vi "TCL Event Viewer.vi"() -> ()   [LabVIEW 2010]
uses:
  <vilib>/Utility/file.llb/Read From Spreadsheet File (string).vi
  TCL Select Fragments/TCL Select Fragments NfragsNcriteria.vi
panel:
  in  "load":bool
  in  "save":bool
  out "event":string
  in  "pick baseline":bool
  in  "auto baseline":bool=TRUE
  in  "load defaults":bool
  in  "calibration constant":dbl=1.0 step=0.0001 format="%#_9f"
  in  "ignore fraction":dbl=0.1875 min=0.0 max=1.0 step=0.0001
  in  "fit fraction":dbl=0.18 min=0.0 max=1.0 step=0.0001
  in  "ignore first":i32=5 min=0 step=1
  in  "subtract fraction":dbl=0.125 min=0.0 max=1.0 step=0.0001
  out "busy":bool
  in  "show all events":bool
  in  "stop":bool
  out "error out":errorcluster
  in  "error in (no error)":errorcluster
  out "polarization %":dbl
  out "area":dbl
  in  "fit order":i32=3 min=0 step=1
  out "fit coefficients":dbl[](array[numeric])
  out "baseline time":timestamp format="%<%H:%M:%S\n%x>T"
  out "baseline":string
  out "raw plot":cluster{dbl[], "signal":dbl[]}[](graph)
  out "poly plot":cluster{dbl[], "poly fit":dbl[]}[](graph)
  out "signal plot":cluster{dbl[], "signal":dbl[]}(graph)
  in  "events list":i32(listbox)
  in  "y axis":string(combo)
  out "events plot":cluster{timestamp, dbl}[](graph)
  out "raw data":string[][](table)
  in  "auto advance":bool
  in  "real time":bool
  in  "end time":timestamp format="%<%H:%M:%S\n%x>T"
  in  "start time":timestamp format="%<%H:%M:%S\n%x>T"
  in  "filter":T1(array[cluster])
  in  "pick baseline files":bool
  in  "use current event file":bool
  in  "pick event files":bool
  in  "additional baseline files":path[](array[path])
  in  "event files":path[](array[path])
  # "Do not operate panel while busy light is on"
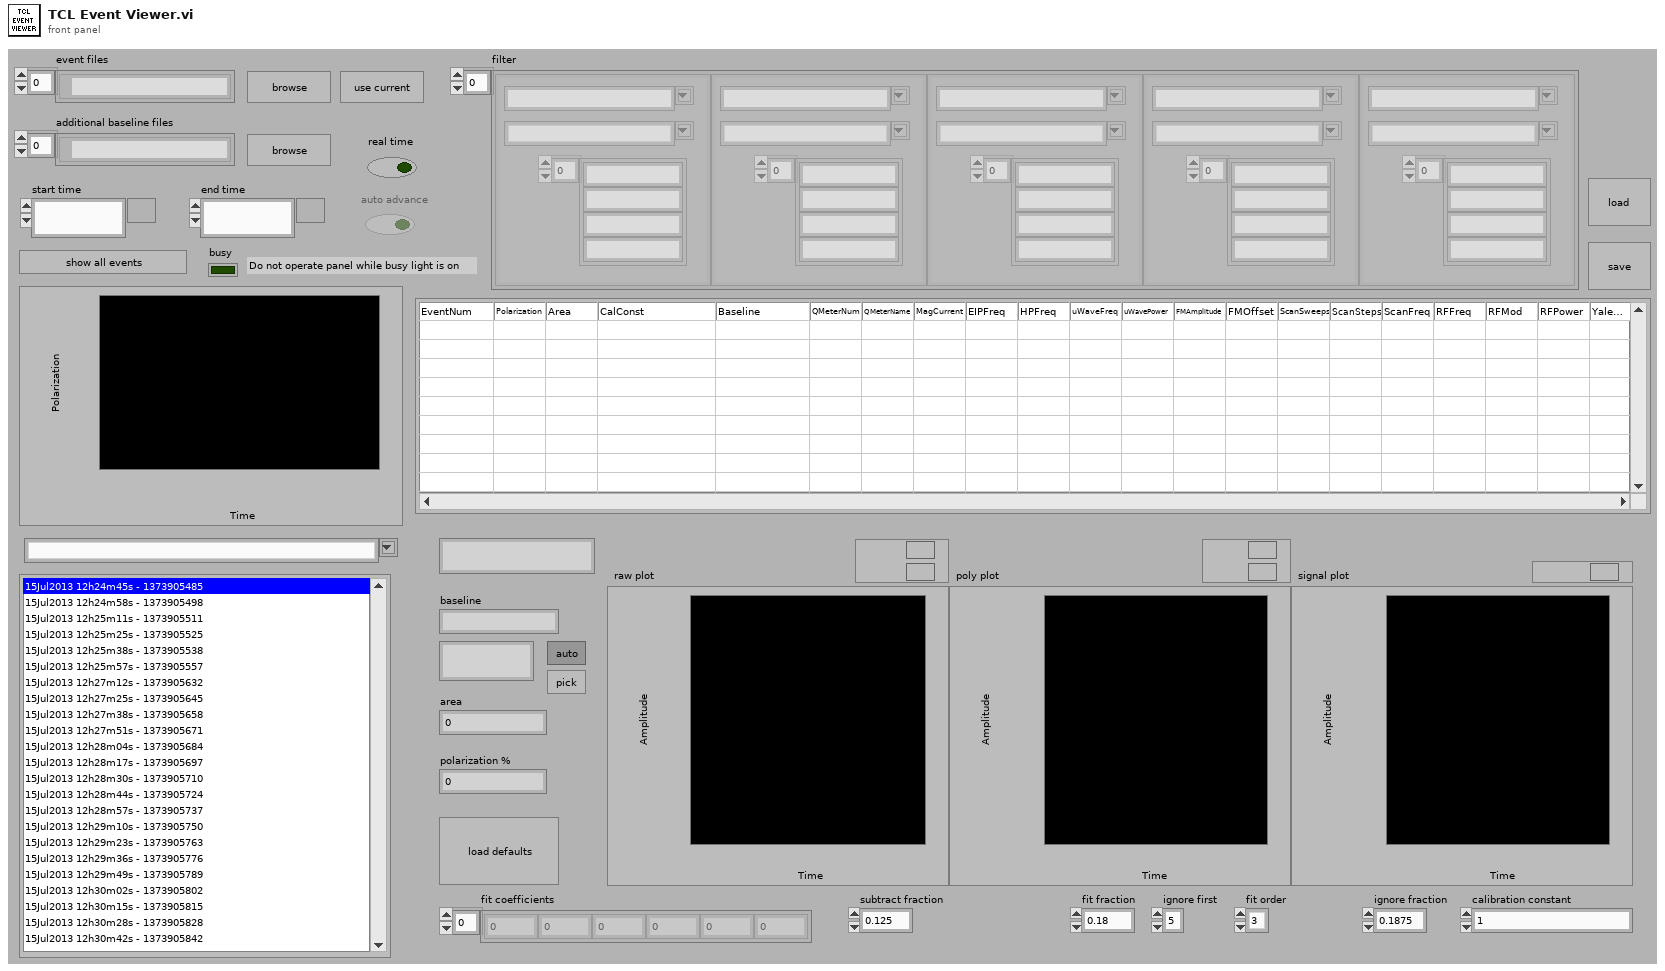
[diagram p1: front panel]
types:
  T1 = cluster{"fragment":string, "criteria":string[], "operator":string}[]
  T2 = enum16{"idle", "import events", "filter events", "plot events", "read plot data", "plot signals"}
  T3 = enum16{"idle", "import events", "filter events", "plot events", "plot signals"}
  T4 = cluster{"primary key":string, "criteria":string[], "operator":string}[]
  T5 = enum16{"big-endian, network order", "native, host order", "little-endian"}
  T6 = cluster{"fragment":string, "criteria":string[], "operator":string}
  T7 = enum8{"Enabled", "Disabled", "Disabled and Grayed Out"}
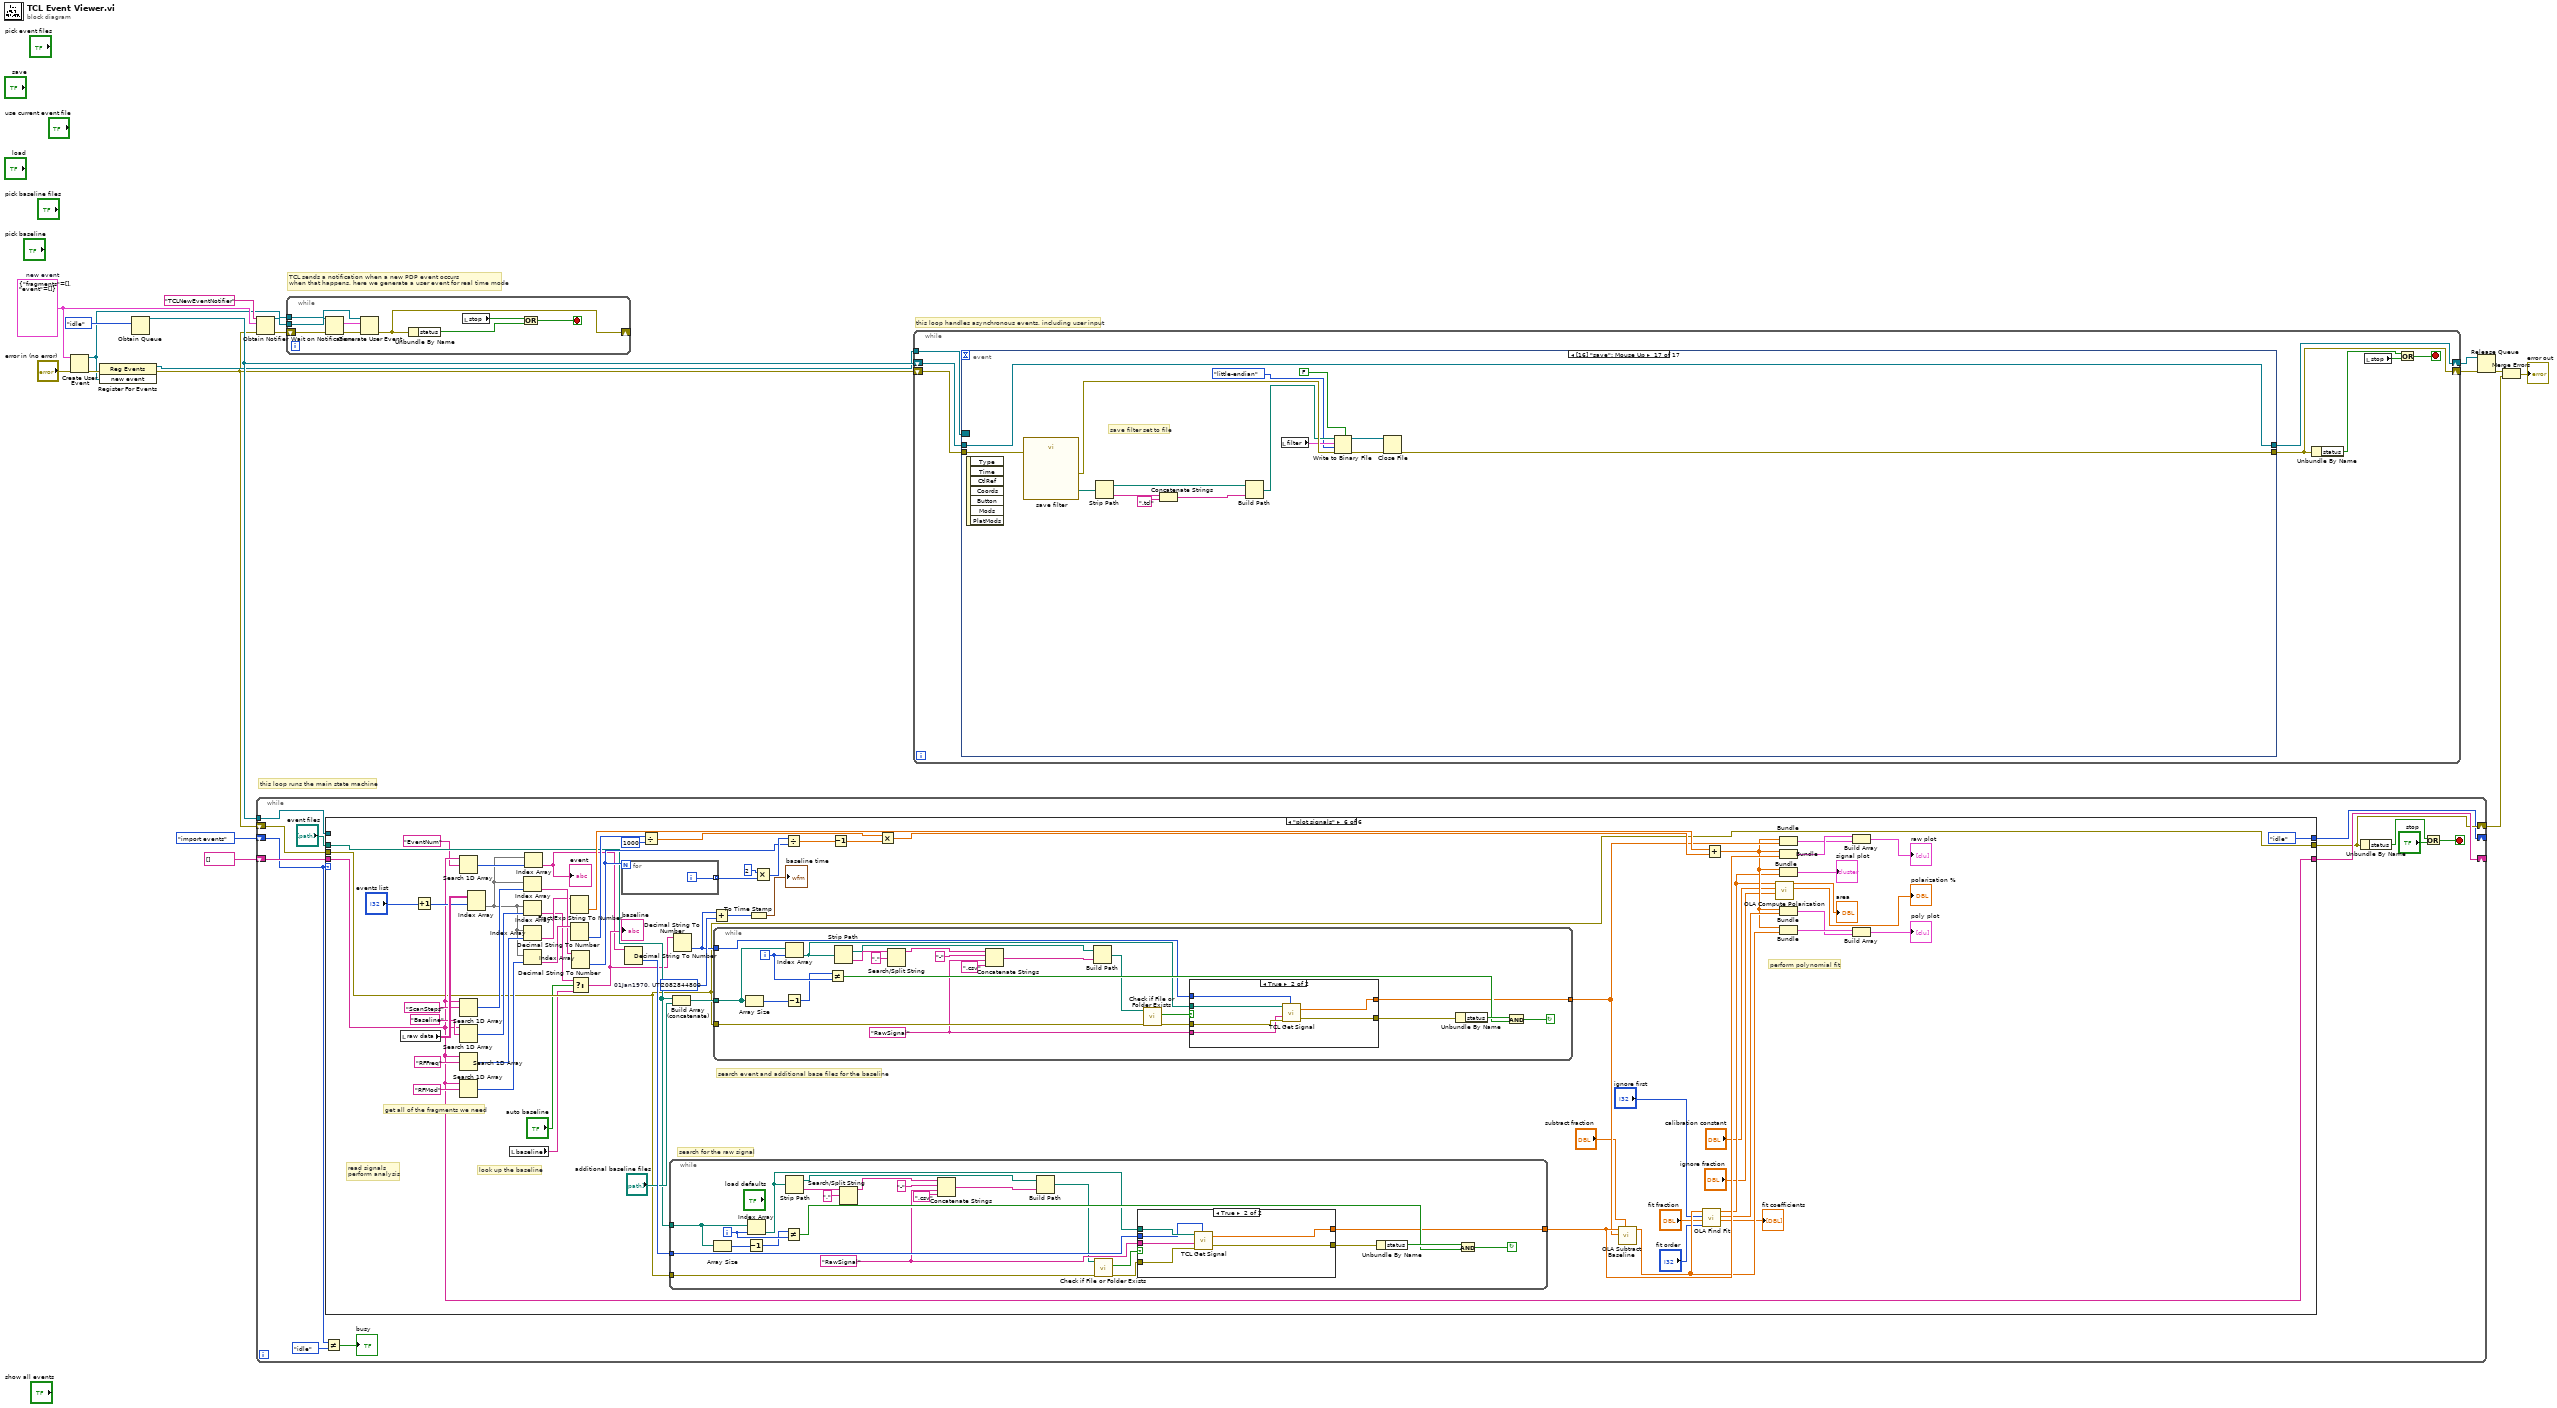
[diagram p0: block diagram]
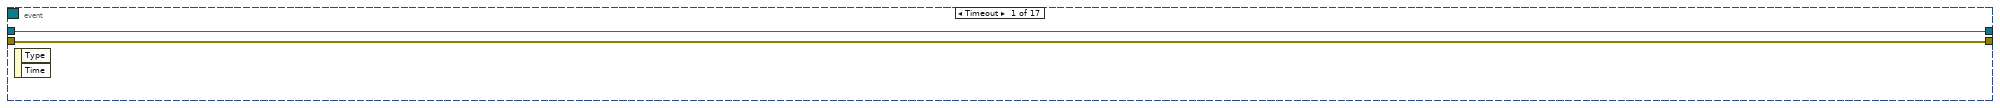
[diagram p2: hidden frame]
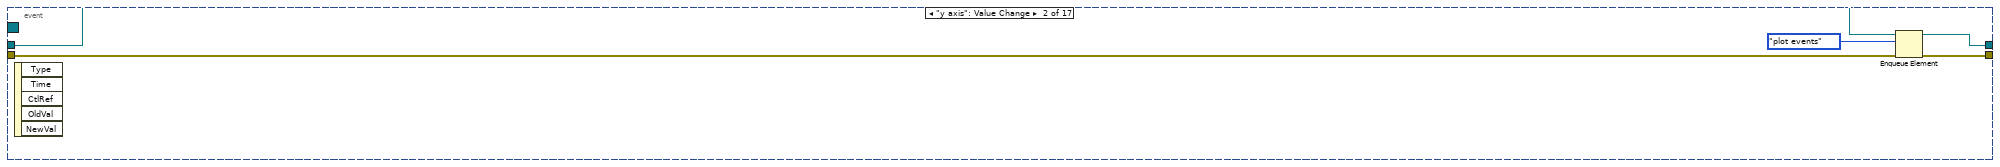
[diagram p3: hidden frame]
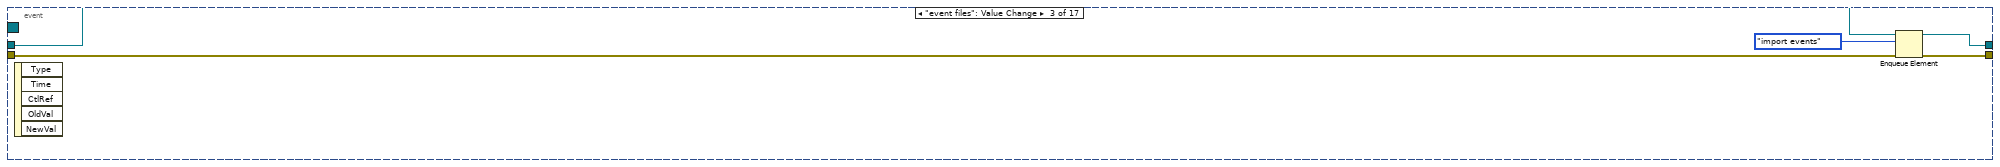
[diagram p4: hidden frame]
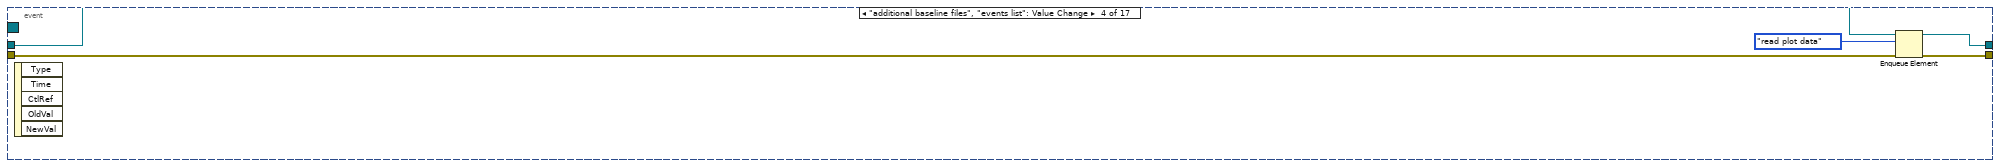
[diagram p5: hidden frame]
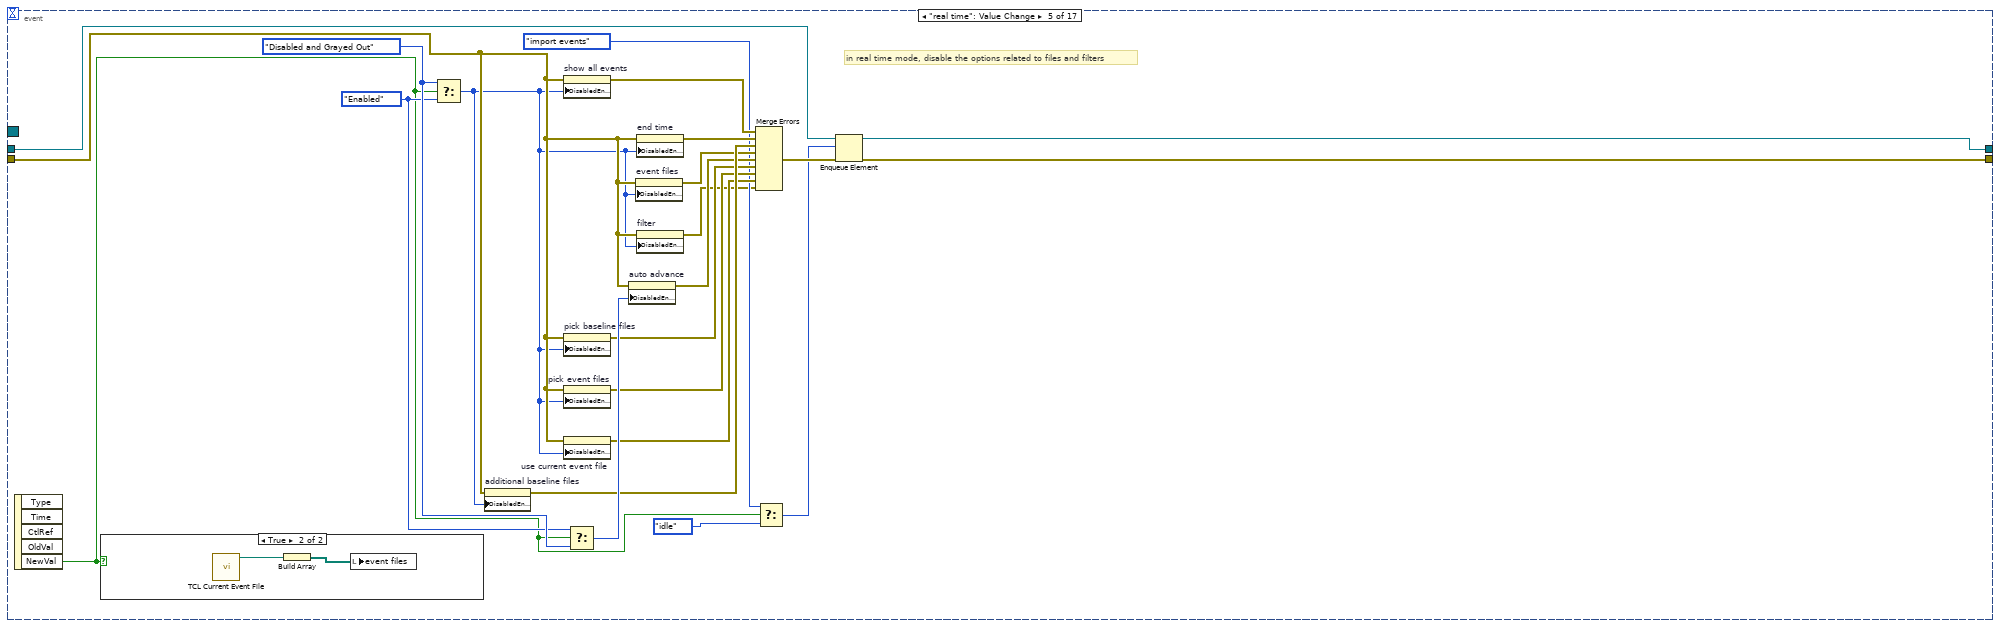
[diagram p6: hidden frame]
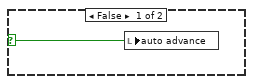
[diagram p7: hidden frame]
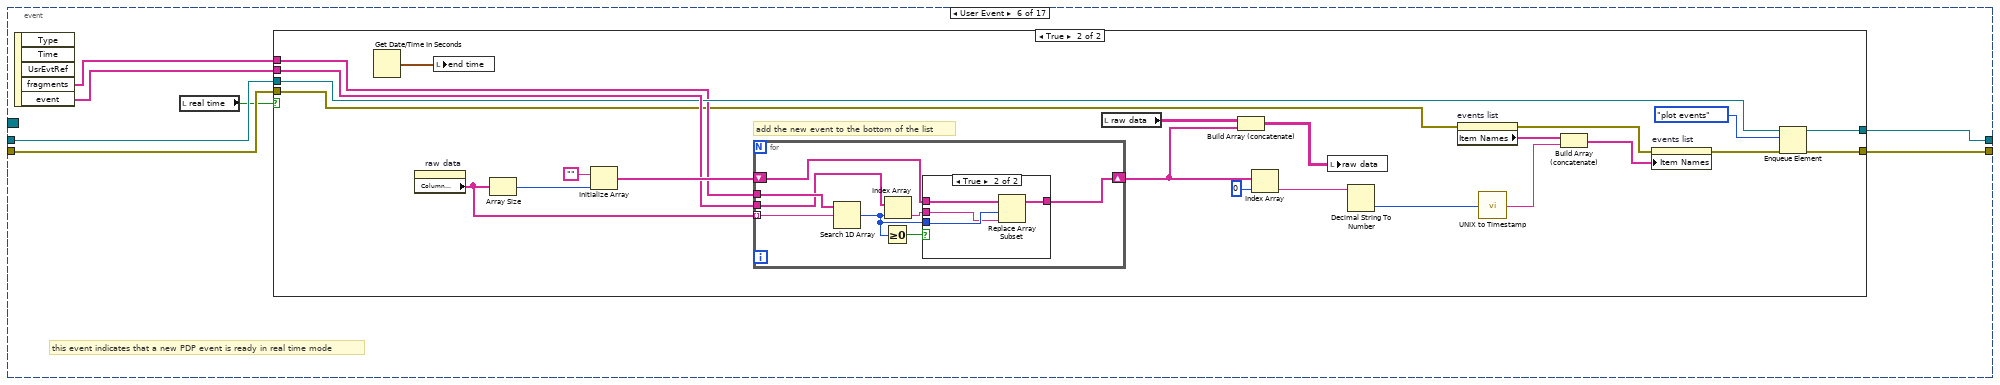
[diagram p8: hidden frame]
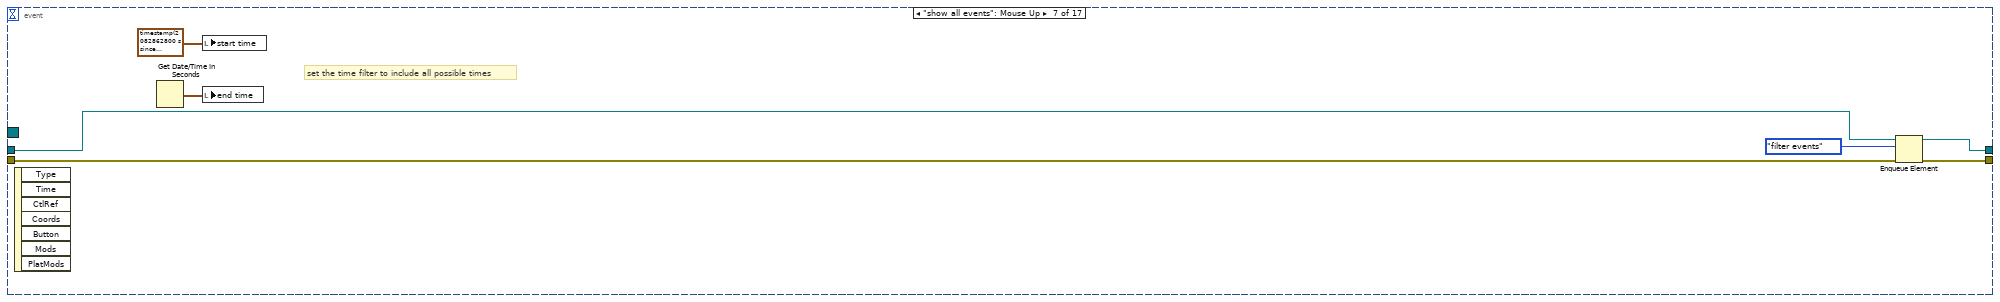
[diagram p11: hidden frame]
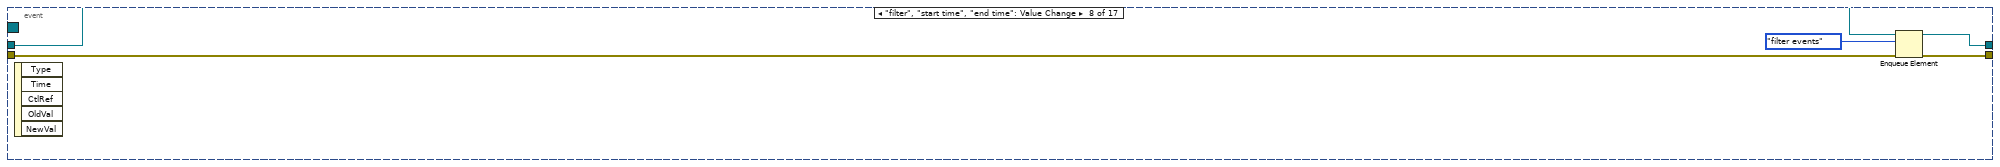
[diagram p12: hidden frame]
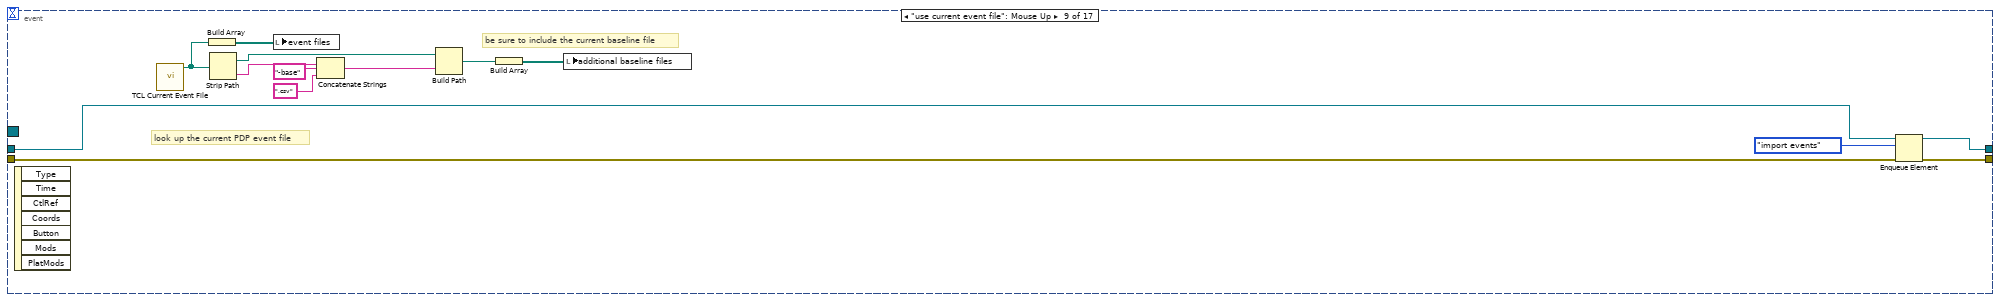
[diagram p13: hidden frame]
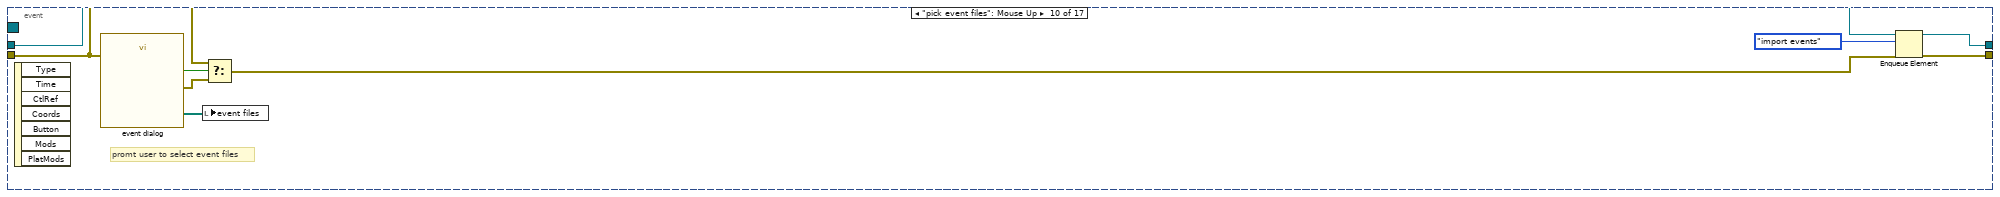
[diagram p14: hidden frame]
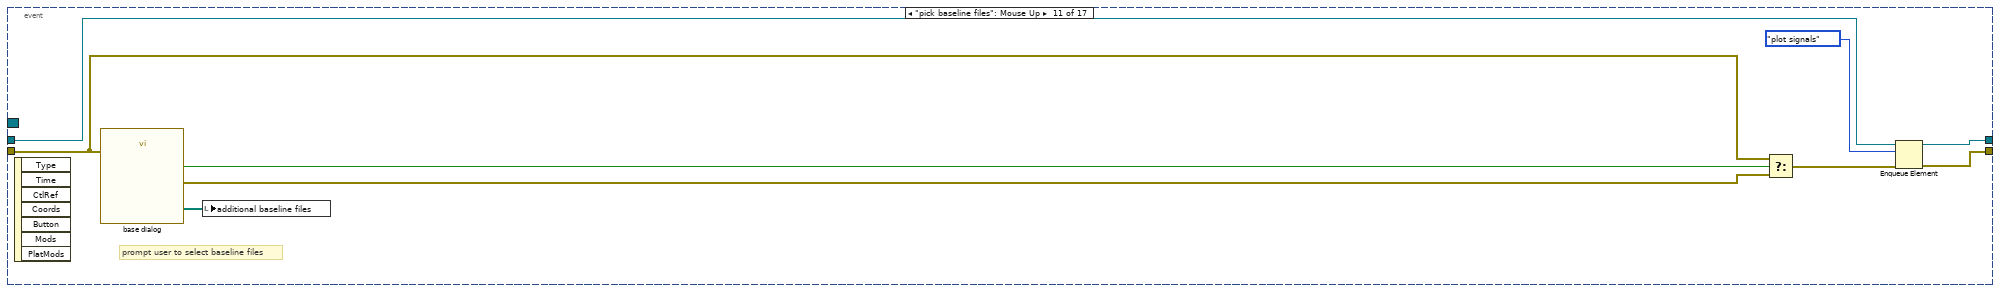
[diagram p15: hidden frame]
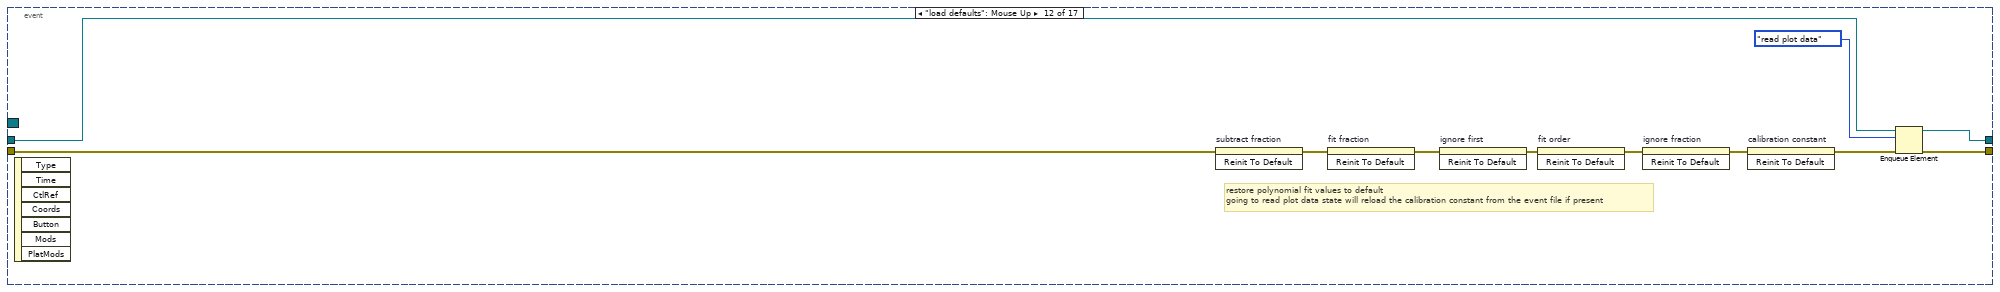
[diagram p16: hidden frame]
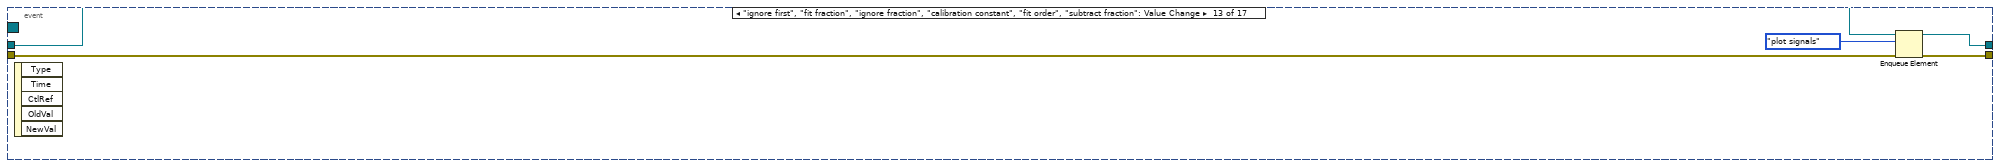
[diagram p17: hidden frame]
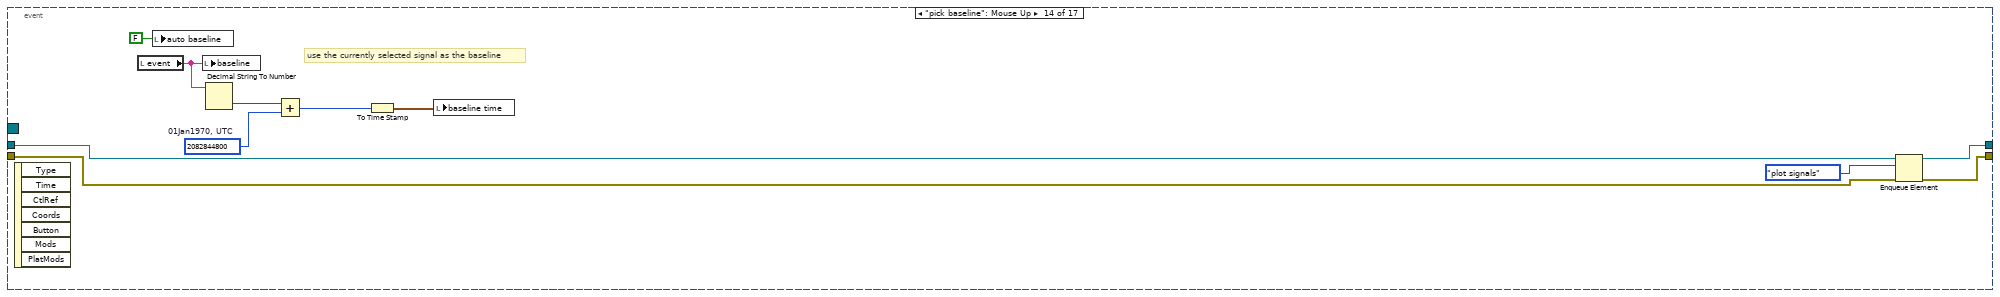
[diagram p18: hidden frame]
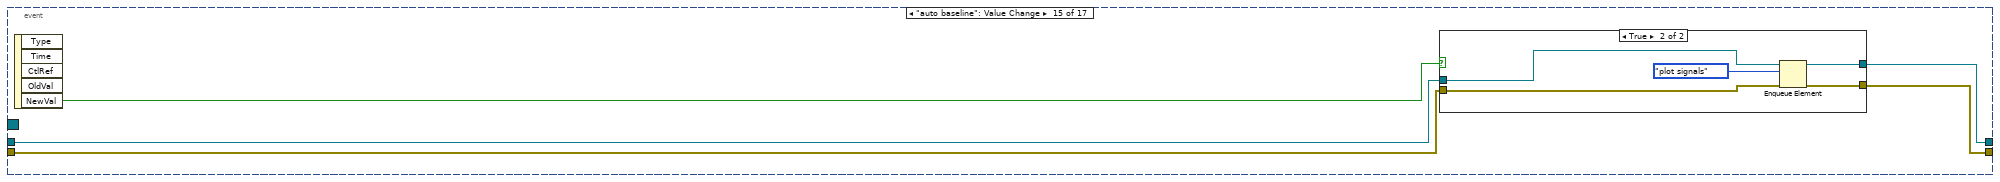
[diagram p19: hidden frame]
diagram:
  w4 = cluster{"fragments":string[], "event":string[]} {"fragments"=[], "event"=[]}  # new event
  # "this loop runs the main state machine"
  # "this loop handles asynchronous events, including user input"
  # "TCL sends a notification when a new PDP event occurs\nwhen that happens, here we generate a user event for real time mode"
  n1 = Create User Event(user event datatype=w4, error in="error in (no error)") -> (user event=w1:refnum<user-event>, error out=w7:errorcluster)
  n2 = register-events(error in=w7, w1) -> (reference out=w9:refnum<event-registration>, error out=w5:errorcluster)  [unwired: 1 in]
  n3 = Obtain Queue(element data type=T2."idle") -> (queue out=w15:refnum<queue>)  [unwired: 4 in, 2 out]
  n4 = Obtain Notifier(name (unnamed)="TCLNewEventNotifier", notification data type=w4, error in (no error)=w5) -> (notifier out=w2:refnum<notifier>, error out=w3:errorcluster)  [unwired: 1 in, 1 out]
  n5 = while {
    shift-right: [w22] -> _
    shift-left: T2."import events" -> [w21]
    shift-right: [w25] -> w11
    shift-left: w5 -> [w29]
    shift-right: [w28] -> _
    shift-left: string[] [] -> [w27]
    tunnel: w15 -> [w23]
    stop <- w31 stop-if-true
    n6 = Not Equal?(x=w21, y=T3."idle") -> (x != y?=→"busy":bool)
    n7 = case shown="\"plot signals\"" w21 {
      tunnel: w29 -> [w33 w51 w91 w143 w190 w226]
      tunnel: [w36 w37 w81 w150 w192 w228] -> w28
      tunnel: [w32 w50 w87 w141 w190 w226] -> w25
      tunnel: [w34 w43 T2."plot events" T2."read plot data" T2."plot signals" T2."idle"] -> w22
      tunnel: w27 -> [w36 _ w81 w150 w192 w228]
      tunnel: "event files" -> [_ w39 w92 _ _ w234]
      tunnel: w23 -> [w35 _ _ _ _ _]
      frame "idle", Default {
        # "do nothing; wait for change of state"
        n8 = Dequeue Element(queue=w35, error in (no error)=w33) -> (element=w34:T2, error out=w32:errorcluster)  [unwired: 1 in, 2 out]
      }
      frame "import events" {
        # "if any event files were selected, start filtering"
        # "reset filters"
        # "loop through all event files"
        # "read events from files"
        n9 = Get Date/Time In Seconds() -> (seconds since 1Jan1904=w46:timestamp)
        n10 = local write "end time"(w46) -> ()
        n11 = for {
          tunnel: w39 -> [w63] mode=indexing
          shift-right: [w52] -> w37
          shift-left: string[] [] -> [w54]
          # "collect all fragments\nfrom all files"
          # "search header for new fragments"
          # "read spreadsheet data"
          n12 = call-poly <vilib>:"Read From Spreadsheet File.vi"("delimiter (\\t)"="," ("delimiter (\\t)"), "number of rows (all:-1)"=1, "file path (dialog if empty)"=w63) -> ("first row"=w60:string[])  [unwired: 4 in, 4 out]
          n13 = Array Size(array=w60) -> (size(s)=w59:i32)
          n14 = Initialize Array("", w59) -> (w57:string[])
          n15 = for {
            tunnel: w60 -> [w67] mode=indexing
            shift-right: [w74] -> w55
            shift-left: 0 -> [w68]
            shift-right: [w73] -> w56
            shift-left: w57 -> [w65]
            tunnel: w54 -> [w72]
            n16 = Increment(x=w68) -> (x+1=w69:i32)
            n17 = Replace Array Subset(array=w65, new element=w67, index=w68) -> (w66:string[])
            n18 = Search 1D Array(1D array=w72, element=w67) -> (index of element=w71:i32)  [unwired: 1 in]
            n19 = Greater Or Equal To 0?(x=w71) -> (x >= 0?=w70:bool)
            n20 = Select(t=w68, s=w70, f=w69) -> (s? t:f=w74:i32)
            n21 = Select(t=w65, s=w70, f=w66) -> (s? t:f=w73:string[])
          }
          n22 = Array Subset(array=w56, length=w55) -> (w53:string[])  [unwired: 1 in]
          n23 = Build Array (concatenate)(w54, w53) -> (w52:string[])
        }
        n24 = Empty Array?(array=w39) -> (empty?=w42:bool)
        n25 = local write "y axis"("EventNum" ("y axis")) -> ()
        n26 = local write "start time"(timestamp(2082862800.2649255 s since 1904-01-01) ("start time")) -> ()
        n27 = Select(t=T2."idle", s=w42, f=T2."filter events") -> (s? t:f=w43:T2)
        n28 = local write "filter"(T1 [] ("filter")) -> ()
        n29 = property on="fragment" class="CmbBox"(error in=w51, "Strings[]"=w37) -> (error out=w49:errorcluster)  [unwired: 1 in, 1 out]
        n30 = property on="y axis" class="CmbBox"(error in=w51, "Strings[]"=w37) -> (error out=w48:errorcluster)  [unwired: 1 in, 1 out]
        n31 = Merge Errors(w49, w48) -> (w50:errorcluster)
      }
      frame "filter events" {
        # "prepare events list for signal selection"
        # "process each file separately"
        # "apply filtering criteria to events"
        n32 = local write "events list"(0 ("events list")) -> ()
        n33 = for {
          tunnel: w92 -> [w101] mode=indexing
          tunnel: w91 -> [w134]
          tunnel: w81 -> [w107]
          tunnel: [w119] -> w80
          shift-right: [w105] -> w82
          shift-left: string[][] [] -> [w103]
          w115 = 2082844800  # 01Jan1970, UTC
          w124 = "EventNum" ("primary key")
          # "map fragments from each file to fragments from all files"
          # "perform SQL select"
          # "add time criteria"
          n34 = To Double Precision Float(number="start time") -> (double precision float=w130:dbl)
          n35 = To Double Precision Float(number="end time") -> (double precision float=w116:dbl)
          n36 = Subtract(x=w130, y=w115) -> (x-y=w118:dbl)
          n37 = Subtract(x=w116, y=w115) -> (x-y=w117:dbl)
          n38 = Number To Decimal String(number=w118) -> (decimal integer string=w129:string)  [unwired: 1 in]
          n39 = Number To Decimal String(number=w117) -> (decimal integer string=w126:string)  [unwired: 1 in]
          n40 = Build Array(w129) -> (w128:string[])
          n41 = Build Array(w126) -> (w125:string[])
          n42 = Bundle("primary key"=w124, w128, "is greater than or equal to") -> (w122:cluster{"primary key":string, string[], string})  [unwired: 1 in]
          n43 = Bundle("primary key"=w124, w125, "is less than or equal to") -> (w121:cluster{"primary key":string, string[], string})  [unwired: 1 in]
          n44 = Build Array (concatenate)("filter", w122, w121) -> (w120:T4)
          n45 = call-poly "TCL Select Fragments.vi"("event file"=w101, "fragments"=w107, "primary key"=w124, "criteria"=w120, "error in (no error)"=w134) -> ("fragments out"=w102:string[], "matches"=w108:string[][], "error out"=w119:errorcluster)  [unwired: 1 in]
          n46 = Array Size(array=w102) -> (size(s)=w109:i32)
          n47 = Array Size(array=w108) -> (size(s)=w112:i32[])
          n48 = Index Array(array=w112, index=0) -> (element=w110:i32)
          n49 = Initialize Array("", w110, w109) -> (w114:string[][])
          n50 = Transpose 2D Array(2D array=w108) -> (transposed array=w106:string[][])
          n51 = for {
            shift-right: [w136] -> w104
            shift-left: w114 -> [w139]
            tunnel: w106 -> [w137] mode=indexing
            tunnel: w107 -> [w140]
            tunnel: w102 -> [w135] mode=indexing
            n52 = Search 1D Array(1D array=w140, element=w135) -> (index of element=w138:i32)  [unwired: 1 in]
            n53 = Replace Array Subset(array=w139, new element=w137, index (col)=w138) -> (w136:string[][])  [unwired: 1 in]
          }
          n54 = Build Array (concatenate)(w103, w104) -> (w105:string[][])
        }
        "raw data" <- w82
        n55 = Array Subset(array=w82, index (row)=1 ("index")) -> (w90:string[][])  [unwired: 3 in]
        n56 = Index Array(array=w90, index (col)=0 ("disabled index (col)")) -> (element=w78:string[])  [unwired: 1 in]
        n57 = Array Size(array=w78) -> (size(s)=w77:i32)
        n58 = Initialize Array("", w77) -> (w76:string[])
        n59 = for {
          tunnel: w78 -> [w96] mode=indexing
          shift-right: [w95] -> w88
          shift-left: w76 -> [w100]
          i -> [w98]
          n60 = Decimal String To Number(string=w96) -> (number=w99:i32)  [unwired: 2 in, 1 out]
          n61 = call "UNIX to Timestamp.vi"("Seconds"=w99) -> ("Timestamp String"=w94:string)
          n62 = Concatenate Strings(w94, " - " ("string"), w96) -> (w93:string)
          n63 = Replace Array Subset(array=w100, new element=w93, index=w98) -> (w95:string[])
        }
        n64 = property on="raw data" class="Tbl (strict)"(error in=w80, "Column Headers[]"=w81) -> (error out=w79:errorcluster)  [unwired: 1 in, 1 out]
        n65 = property on="events list" class="LstBox (strict)"(error in=w79, "Item Names"=w88) -> (error out=w87:errorcluster)  [unwired: 1 in, 1 out]
      }
      frame "plot events" {
        w156 = u64 2082844800  # 01Jan1970, UTC
        # "in auto advance mode, choose the latest event"
        # "find the y axis"
        # "plot events on the custom graph"
        n66 = local read "raw data"() -> (w151:string[][])
        n67 = Search 1D Array(1D array=w150, element="y axis") -> (index of element=w159:i32)  [unwired: 1 in]
        n68 = Search 1D Array(1D array=w150, element="EventNum") -> (index of element=w161:i32)  [unwired: 1 in]
        n69 = Array Subset(array=w151, index (row)=1 ("index")) -> (w160:string[][])  [unwired: 3 in]
        n70 = Index Array(array=w160, index (col)=w159) -> (element=w153:string[])  [unwired: 1 in]
        n71 = Index Array(array=w160, index (col)=w161) -> (element=w158:string[])  [unwired: 1 in]
        n72 = Decimal String To Number(string=w158) -> (number=w157:i32[])  [unwired: 2 in, 1 out]
        n73 = Add(x=w157, y=w156) -> (x+y=w155:u64[])
        n74 = Fract/Exp String To Number(string=w153) -> (number=w147:dbl[])  [unwired: 3 in, 1 out]
        n75 = To Time Stamp(1:w155) -> (0:w154:timestamp[])
        n76 = Array Size(array=w147) -> (size(s)=w146:i32)
        n77 = Build Cluster Array(w154, w147) -> (→"events plot":cluster{timestamp, dbl}[])
        n78 = Decrement(x=w146) -> (x-1=w145:i32)
        n79 = case shown="True" "auto advance" {
          tunnel: w145 -> [w164 _]
          tunnel: w143 -> [w165 w180]
          tunnel: [w172 w177] -> w142
          frame True {
            n80 = local write "events list"(w164) -> ()
            n81 = Subtract(x=w164, y=u32 7) -> (x-y=w167:u32)
            n82 = Subtract(x=w164, y=22) -> (x-y=w176:i32)
            n83 = Bundle(w167, "y"=u32 0) -> (w170:cluster{u32, "y":u32})  [unwired: 1 in]
            n84 = property on="raw data" class="Tbl (strict)"(error in=w165, "Index Values"=w170) -> (error out=w169:errorcluster)  [unwired: 1 in, 1 out]
            n85 = Max & Min(x=w176, y=0) -> (max(x,y)=w171:i32)  [unwired: 1 out]
            n86 = property on="events list" class="LstBox (strict)"(error in=w169, "Key Focus"=TRUE, "Top Row"=w171) -> (error out=w172:errorcluster)  [unwired: 1 in, 1 out]
          }
          frame False {
            n87 = property on="events list" class="LstBox (strict)"(error in=w180, "Key Focus"=TRUE) -> (error out=w178:errorcluster)  [unwired: 1 in, 1 out]
            n88 = case shown="True" "real time" {
              tunnel: w178 -> [w182 w185]
              tunnel: [w182 w184] -> w177
              frame True {
              }
              frame False {
                w183 = 0 ("Active Row:Active Row Number")
                n89 = property on="events list" class="LstBox (strict)"(error in=w185, "Active Row"=w183, "Top Row"=w183) -> (error out=w184:errorcluster)  [unwired: 1 in, 1 out]
              }
            }
          }
        }
        n90 = property on="events plot" class="XYGraph (strict)"(error in=w142, "YScale.NameLbl.Text"="y axis") -> (error out=w141:errorcluster)  [unwired: 1 in, 1 out]
      }
      frame "read plot data" {
        # "read variables necessary for polynomial fit"
        n91 = local read "events list"() -> (w200:i32)
        n92 = local read "raw data"() -> (w198:string[][])
        n93 = Increment(x=w200) -> (x+1=w199:i32)
        n94 = Search 1D Array(1D array=w192, element="CalConst") -> (index of element=w195:i32)  [unwired: 1 in]
        n95 = Index Array(array=w198, index (row)=w199) -> (element=w196:string[])  [unwired: 1 in]
        n96 = Index Array(array=w196, index=w195) -> (element=w194:string)
        n97 = local read "calibration constant"() -> (w186:dbl)
        n98 = Fract/Exp String To Number(string=w194) -> (offset past number=w188:i32, number=w193:dbl)  [unwired: 3 in]
        n99 = Not Equal To 0?(x=w188) -> (x != 0?=w187:bool)
        n100 = Select(t=w193, s=w187, f=w186) -> (s? t:f=w189:dbl)
        n101 = local write "calibration constant"(w189) -> ()
      }
      frame "plot signals" {
        w233 = u64 2082844800  # 01Jan1970, UTC
        # "perform polynomial fit"
        # "search for the raw signal"
        # "search event and additional base files for the baseline"
        # "look up the baseline"
        # "get all of the fragments we need"
        # "read signals\nperform analysis"
        n102 = local read "raw data"() -> (w266:string[][])
        n103 = Increment(x="events list") -> (x+1=w265:i32)
        n104 = Search 1D Array(1D array=w228, element="EventNum") -> (index of element=w243:i32)  [unwired: 1 in]
        n105 = Search 1D Array(1D array=w228, element="ScanSteps") -> (index of element=w258:i32)  [unwired: 1 in]
        n106 = Search 1D Array(1D array=w228, element="Baseline") -> (index of element=w241:i32)  [unwired: 1 in]
        n107 = Search 1D Array(1D array=w228, element="RFFreq") -> (index of element=w260:i32)  [unwired: 1 in]
        n108 = Search 1D Array(1D array=w228, element="RFMod") -> (index of element=w259:i32)  [unwired: 1 in]
        n109 = Index Array(array=w266, index (row)=w265) -> (element=w229:string[])  [unwired: 1 in]
        n110 = local read "baseline"() -> (w203:string)
        n111 = Index Array(array=w229, index=w258) -> (element=w256:string)
        n112 = Index Array(array=w229, index=w241) -> (element=w205:string)
        n113 = Index Array(array=w229, index=w260) -> (element=w255:string)
        n114 = Index Array(array=w229, index=w259) -> (element=w257:string)
        n115 = Index Array(array=w229, index=w243) -> (element=w201:string)
        "event" <- w201
        n116 = Fract/Exp String To Number(string=w255) -> (number=w244:dbl)  [unwired: 3 in, 1 out]
        n117 = Decimal String To Number(string=w257) -> (number=w249:i32)  [unwired: 2 in, 1 out]
        n118 = Decimal String To Number(string=w256) -> (number=w251:i32)  [unwired: 2 in, 1 out]
        n119 = Select(t=w205, s="auto baseline", f=w203) -> (s? t:f=w206:string)
        "baseline" <- w206
        n120 = for {
          N: w251 -> [_]
          tunnel: [w333] -> w254 mode=indexing
          i -> [w333]
        }
        n121 = Decimal String To Number(string=w201) -> (number=w242:i32)  [unwired: 2 in, 1 out]
        n122 = Divide(x=w249, y=1000) -> (x/y=w246:dbl)
        n123 = while {
          tunnel: w234 -> [w318]
          tunnel: w226 -> [w311]
          tunnel: w242 -> [w314]
          tunnel: [w313] -> w225
          i -> [w319]
          stop <- w321 continue-if-true
          w307 = "RawSignal" ("signal name")
          n124 = Array Size(array=w318) -> (size(s)=w316:i32)
          n125 = Decrement(x=w316) -> (x-1=w317:i32)
          n126 = Index Array(array=w318, index=w319) -> (element=w300:path)
          n127 = Not Equal?(x=w317, y=w319) -> (x != y?=w320:bool)
          n128 = Strip Path(path=w300) -> (stripped path=w302:path, name=w309:string)
          n129 = Search/Split String(string=w309, search string/char (-)=".") -> (substring before match=w303:string)  [unwired: 1 in, 2 out]
          n130 = Concatenate Strings(w303, "-" ("string"), w307, ".csv" ("string")) -> (w305:string)
          n131 = Build Path(base path=w302, name or relative path=w305) -> (appended path=w301:path)
          n132 = call <vilib>:"Check if File or Folder Exists.vi"("error in (no error)"=w311, "path"=w301) -> ("error out"=w310:errorcluster, "file or folder exists?"=w304:bool)  [unwired: 7 in, 1 out]
          n133 = case shown="True" w304 {
            tunnel: w310 -> [w324 w332]
            tunnel: w300 -> [_ w331]
            tunnel: w314 -> [_ w330]
            tunnel: w307 -> [_ w329]
            tunnel: [dbl[] [] ("signal") w328] -> w313
            tunnel: [w325 w327] -> w312
            frame False {
              n134 = call <vilib>:"Error Cluster From Error Code.vi"("error in (no error)"=w324, "error code (0)"=15) -> ("error out"=w325:errorcluster)  [unwired: 7 in]
            }
            frame True {
              n135 = call "TCL Get Signal.vi"("event number"=w330, "error in (no error)"=w332, "signal name"=w329, "event file"=w331) -> ("error out"=w327:errorcluster, "signal"=w328:dbl[])  [unwired: 2 in]
            }
          }
          n136 = Unbundle By Name(w312) -> ("status"=w322:bool)
          n137 = And(x=w322, y=w320) -> (x .and. y?=w321:bool)
        }
        n138 = Build Array (concatenate)(w234, "additional baseline files") -> (w236:path[])
        n139 = Decimal String To Number(string=w206) -> (number=w231:i32)  [unwired: 2 in, 1 out]
        n140 = Add(x=w231, y=w233) -> (x+y=w232:u64)
        n141 = while {
          tunnel: w236 -> [w285]
          tunnel: w226 -> [w277]
          tunnel: w231 -> [w280]
          tunnel: [w279] -> w224
          i -> [w286]
          stop <- w288 continue-if-true
          w272 = "RawSignal" ("signal name")
          n142 = Array Size(array=w285) -> (size(s)=w283:i32)
          n143 = Decrement(x=w283) -> (x-1=w284:i32)
          n144 = Index Array(array=w285, index=w286) -> (element=w267:path)
          n145 = Not Equal?(x=w284, y=w286) -> (x != y?=w287:bool)
          n146 = Strip Path(path=w267) -> (stripped path=w275:path, name=w282:string)
          n147 = Search/Split String(string=w282, search string/char (-)=".") -> (substring before match=w270:string)  [unwired: 1 in, 2 out]
          n148 = Concatenate Strings(w270, "-" ("string"), w272, ".csv" ("string")) -> (w274:string)
          n149 = Build Path(base path=w275, name or relative path=w274) -> (appended path=w268:path)
          n150 = call <vilib>:"Check if File or Folder Exists.vi"("error in (no error)"=w277, "path"=w268) -> ("error out"=w276:errorcluster, "file or folder exists?"=w269:bool)  [unwired: 7 in, 1 out]
          n151 = case shown="True" w269 {
            tunnel: w276 -> [w290 w299]
            tunnel: w267 -> [_ w298]
            tunnel: w280 -> [_ w297]
            tunnel: w272 -> [_ w296]
            tunnel: [dbl[] [] ("signal") w295] -> w279
            tunnel: [w291 w294] -> w278
            frame False {
              n152 = call <vilib>:"Error Cluster From Error Code.vi"("error in (no error)"=w290, "error code (0)"=15) -> ("error out"=w291:errorcluster)  [unwired: 7 in]
            }
            frame True {
              n153 = call "TCL Get Signal.vi"("event number"=w297, "error in (no error)"=w299, "signal name"=w296, "event file"=w298) -> ("error out"=w294:errorcluster, "signal"=w295:dbl[])  [unwired: 2 in]
            }
          }
          n154 = Unbundle By Name(w278) -> ("status"=w289:bool)
          n155 = And(x=w289, y=w287) -> (x .and. y?=w288:bool)
        }
        n156 = To Time Stamp(1:w232) -> (0:→"baseline time":timestamp)
        n157 = Multiply(x=2, y=w254) -> (x*y=w252:i32[])
        n158 = Divide(x=w252, y=w251) -> (x/y=w250:dbl[])
        n159 = Decrement(x=w250) -> (x-1=w247:dbl[])
        n160 = Multiply(x=w246, y=w247) -> (x*y=w245:dbl[])
        n161 = call "OLA Subtract Baseline.vi"("subtract fraction"="subtract fraction", "baseline"=w224, "raw"=w225) -> ("subtracted"=w221:dbl[])  [unwired: 8 in]
        n162 = call "OLA Find Fit.vi"("order"="fit order", "fit fraction"="fit fraction", "ignore first"="ignore first", "signal"=w221) -> ("coefficients"=→"fit coefficients":dbl[], "fit"=w217:dbl[], "subtracted"=w211:dbl[])  [unwired: 5 in]
        n163 = Add(x=w244, y=w245) -> (x+y=w213:dbl[])
        n164 = call "OLA Compute Polarization.vi"("ignore fraction"="ignore fraction", "cal"="calibration constant", "signal"=w211) -> ("polarization"=→"polarization %":dbl, "area"=→"area":dbl)  [unwired: 7 in]
        n165 = Bundle(w213, "signal"=w224) -> (w237:cluster{dbl[], "signal":dbl[]})  [unwired: 1 in]
        n166 = Bundle(w213, "signal"=w225) -> (w238:cluster{dbl[], "signal":dbl[]})  [unwired: 1 in]
        n167 = Bundle(w213, "subtracted"=w211) -> (→"signal plot":cluster{dbl[], "subtracted":dbl[]})  [unwired: 1 in]
        n168 = Bundle(w213, "fit"=w217) -> (w216:cluster{dbl[], "fit":dbl[]})  [unwired: 1 in]
        n169 = Bundle(w213, "subtracted"=w221) -> (w222:cluster{dbl[], "subtracted":dbl[]})  [unwired: 1 in]
        n170 = Build Array(w238, w237) -> (→"raw plot":cluster{dbl[], "signal":dbl[]}[])
        n171 = Build Array(w222, w216) -> (→"poly plot":cluster{dbl[], "fit":dbl[]}[])
      }
    }
    n172 = Unbundle By Name(w25) -> ("status"=w24:bool)
    n173 = Or(x=w24, y="stop") -> (x .or. y?=w31:bool)
  }
  n174 = while {
    shift-right: [w337] -> _
    shift-left: w3 -> [w341]
    tunnel: w2 -> [w342]
    tunnel: w1 -> [w338]
    stop <- w335 stop-if-true
    n175 = Wait on Notification(notifier=w342, error in (no error)=w341) -> (notification=w339:cluster{"fragments":string[], "event":string[]}, error out=w340:errorcluster)  [unwired: 2 in, 2 out]
    n176 = Generate User Event(user event=w338, event data cluster=w339, error in=w340) -> (error out=w337:errorcluster)  [unwired: 1 out]
    n177 = Unbundle By Name(w337) -> ("status"=w336:bool)
    n178 = local read "stop"() -> (w334:bool)
    n179 = Or(x=w334, y=w336) -> (x .or. y?=w335:bool)
  }
  n180 = while {
    shift-right: [w347] -> w14
    shift-left: w15 -> [w346]
    shift-right: [w348] -> w13
    shift-left: w5 -> [w350]
    tunnel: w9 -> [w345]
    stop <- w344 stop-if-true
    n181 = event shown="[16] \"save\": Mouse Up" {
      selector: w345 -> [_ _ _ _ _ _ _ _ _ _ _ _ _ _ _ _ _]
      dyn-events: _ -> [_ _ _ _ _ _ _ _ _ _ _ _ _ _ _ _ _]
      timeout: _ -> [_ _ _ _ _ _ _ _ _ _ _ _ _ _ _ _ _]
      tunnel: [w352 w356 w358 w363 w376 w398 w440 w447 w459 w468 w477 w483 w496 w498 w509 w527 w545] -> w348
      tunnel: w350 -> [w352 w353 w359 w364 w370 w394 w441 w448 w460 w465 w474 w487 w495 w499 w512 w536 w551]
      tunnel: [w351 w355 w362 w367 w374 w396 w444 w446 w463 w472 w481 w482 w497 w502 w510 w530 w544] -> w347
      tunnel: w346 -> [w351 w354 w361 w366 w375 w397 w443 w445 w462 w471 w480 w486 w494 w501 w511 w531 w544]
      event Timeout {
        n182 = event-data() -> ()  [unwired: 1 in, 2 out]
      }
      event "y axis": Value Change {
        n183 = event-data() -> ()  [unwired: 1 in, 5 out]
        n184 = Enqueue Element(queue=w354, element=T2."plot events", error in (no error)=w353) -> (queue out=w355:refnum<queue>, error out=w356:errorcluster)  [unwired: 1 in, 1 out]
      }
      event "event files": Value Change {
        n185 = event-data() -> ()  [unwired: 1 in, 5 out]
        n186 = Enqueue Element(queue=w361, element=T2."import events", error in (no error)=w359) -> (queue out=w362:refnum<queue>, error out=w358:errorcluster)  [unwired: 1 in, 1 out]
      }
      event "additional baseline files", "events list": Value Change {
        n187 = event-data() -> ()  [unwired: 1 in, 5 out]
        n188 = Enqueue Element(queue=w366, element=T2."read plot data", error in (no error)=w364) -> (queue out=w367:refnum<queue>, error out=w363:errorcluster)  [unwired: 1 in, 1 out]
      }
      event "real time": Value Change {
        w387 = T7."Enabled" ("Disabled")
        w388 = T7."Disabled and Grayed Out" ("Disabled")
        # "in real time mode, disable the options related to files and filters"
        n189 = event-data() -> ("NewVal"=w372:bool)  [unwired: 1 in, 4 out]
        n190 = case shown="True" w372 {
          selector: w372 -> [w390 _]
          frame False {
            n191 = local write "auto advance"(w390) -> ()
          }
          frame True {
            n192 = call "TCL Current Event File.vi"() -> ("current event file"=w391:path)  [unwired: 11 in]
            n193 = Build Array(w391) -> (w392:path[])
            n194 = local write "event files"(w392) -> ()
          }
        }
        n195 = Select(t=w388, s=w372, f=w387) -> (s? t:f=w369:T7)
        n196 = property on="additional baseline files" class="Arr (strict)"(error in=w370, "DisabledEnum"=w369) -> (error out=w384:errorcluster)  [unwired: 1 in, 1 out]
        n197 = property on="show all events" class="Bool (strict)"(error in=w370, "DisabledEnum"=w369) -> (error out=w386:errorcluster)  [unwired: 1 in, 1 out]
        n198 = property on="pick baseline files" class="Bool (strict)"(error in=w370, "DisabledEnum"=w369) -> (error out=w381:errorcluster)  [unwired: 1 in, 1 out]
        n199 = property on="pick event files" class="Bool (strict)"(error in=w370, "DisabledEnum"=w369) -> (error out=w380:errorcluster)  [unwired: 1 in, 1 out]
        n200 = property on="use current event file" class="Bool (strict)"(error in=w370, "DisabledEnum"=w369) -> (error out=w379:errorcluster)  [unwired: 1 in, 1 out]
        n201 = Select(t=w387, s=w372, f=w388) -> (s? t:f=w389:T7)
        n202 = property on="auto advance" class="Bool (strict)"(error in=w370, "DisabledEnum"=w389) -> (error out=w382:errorcluster)  [unwired: 1 in, 1 out]
        n203 = property on="event files" class="Arr (strict)"(error in=w370, "DisabledEnum"=w369) -> (error out=w383:errorcluster)  [unwired: 1 in, 1 out]
        n204 = property on="end time" class="AbsTime (strict)"(error in=w370, "DisabledEnum"=w369) -> (error out=w385:errorcluster)  [unwired: 1 in, 1 out]
        n205 = property on="filter" class="Arr (strict)"(error in=w370, "DisabledEnum"=w369) -> (error out=w368:errorcluster)  [unwired: 1 in, 1 out]
        n206 = Merge Errors(w386, w385, w384, w383, w382, w381, w380, w379, w368) -> (w377:errorcluster)
        n207 = Select(t=T2."import events" ("element"), s=w372, f=T2."idle" ("element")) -> (s? t:f=w373:T2)
        n208 = Enqueue Element(queue=w375, element=w373, error in (no error)=w377) -> (queue out=w374:refnum<queue>, error out=w376:errorcluster)  [unwired: 1 in, 1 out]
      }
      event User Event {
        # "this event indicates that a new PDP event is ready in real time mode"
        n209 = event-data() -> ("fragments"=w395:string[], "event"=w399:string[])  [unwired: 1 in, 3 out]
        n210 = local read "real time"() -> (w393:bool)
        n211 = case shown="True" w393 {
          tunnel: w399 -> [_ w421]
          tunnel: [w400 w417] -> w398
          tunnel: w397 -> [w401 w416]
          tunnel: [w401 w415] -> w396
          tunnel: w395 -> [_ w413]
          tunnel: w394 -> [w400 w404]
          frame False {
          }
          frame True {
            # "add the new event to the bottom of the list"
            n212 = Get Date/Time In Seconds() -> (seconds since 1Jan1904=w414:timestamp)
            n213 = property on="raw data" class="Tbl (strict)"() -> ("Column Headers[]"=w402:string[])  [unwired: 2 in, 2 out]
            n214 = local write "end time"(w414) -> ()
            n215 = Array Size(array=w402) -> (size(s)=w424:i32)
            n216 = Initialize Array("", w424) -> (w422:string[])
            n217 = for {
              tunnel: w402 -> [w431] mode=indexing
              tunnel: w413 -> [w432]
              tunnel: w421 -> [w430]
              shift-right: [w425] -> w411
              shift-left: w422 -> [w427]
              n218 = Search 1D Array(1D array=w432, element=w431) -> (index of element=w429:i32)  [unwired: 1 in]
              n219 = Greater Or Equal To 0?(x=w429) -> (x >= 0?=w428:bool)
              n220 = Index Array(array=w430, index=w429) -> (element=w426:string)
              n221 = case shown="True" w428 {
                tunnel: w429 -> [_ w437]
                tunnel: w427 -> [w433 w436]
                tunnel: w426 -> [_ w435]
                tunnel: [w433 w434] -> w425
                frame False {
                }
                frame True {
                  n222 = Replace Array Subset(array=w436, new element=w435, index=w437) -> (w434:string[])
                }
              }
            }
            n223 = local read "raw data"() -> (w420:string[][])
            n224 = Build Array (concatenate)(w420, w411) -> (w419:string[][])
            n225 = Index Array(array=w411, index=0) -> (element=w410:string)
            n226 = local write "raw data"(w419) -> ()
            n227 = Decimal String To Number(string=w410) -> (number=w408:i32)  [unwired: 2 in, 1 out]
            n228 = property on="events list" class="LstBox (strict)"(error in=w404) -> (error out=w405:errorcluster, "Item Names"=w412:string[])  [unwired: 1 in, 1 out]
            n229 = call "UNIX to Timestamp.vi"("Seconds"=w408) -> ("Timestamp String"=w407:string)
            n230 = Build Array (concatenate)(w412, w407) -> (w406:string[])
            n231 = property on="events list" class="LstBox (strict)"(error in=w405, "Item Names"=w406) -> (error out=w403:errorcluster)  [unwired: 1 in, 1 out]
            n232 = Enqueue Element(queue=w416, element=T2."plot events", error in (no error)=w403) -> (queue out=w415:refnum<queue>, error out=w417:errorcluster)  [unwired: 1 in, 1 out]
          }
        }
      }
      event "show all events": Mouse Up {
        # "set the time filter to include all possible times"
        n233 = event-data() -> ()  [unwired: 1 in, 7 out]
        n234 = Get Date/Time In Seconds() -> (seconds since 1Jan1904=w438:timestamp)
        n235 = local write "start time"(timestamp(2082862800.2649255 s since 1904-01-01) ("start time")) -> ()
        n236 = local write "end time"(w438) -> ()
        n237 = Enqueue Element(queue=w443, element=T2."filter events", error in (no error)=w441) -> (queue out=w444:refnum<queue>, error out=w440:errorcluster)  [unwired: 1 in, 1 out]
      }
      event "filter", "start time", "end time": Value Change {
        n238 = event-data() -> ()  [unwired: 1 in, 5 out]
        n239 = Enqueue Element(queue=w445, element=T2."filter events", error in (no error)=w448) -> (queue out=w446:refnum<queue>, error out=w447:errorcluster)  [unwired: 1 in, 1 out]
      }
      event "use current event file": Mouse Up {
        # "be sure to include the current baseline file"
        # "look up the current PDP event file"
        n240 = event-data() -> ()  [unwired: 1 in, 7 out]
        n241 = call "TCL Current Event File.vi"() -> ("current event file"=w452:path)  [unwired: 11 in]
        n242 = Build Array(w452) -> (w458:path[])
        n243 = Strip Path(path=w452) -> (stripped path=w450:path, name=w451:string)
        n244 = local write "event files"(w458) -> ()
        n245 = Concatenate Strings(w451, "-base" ("string"), ".csv" ("string")) -> (w455:string)
        n246 = Build Path(base path=w450, name or relative path=w455) -> (appended path=w454:path)
        n247 = Build Array(w454) -> (w453:path[])
        n248 = local write "additional baseline files"(w453) -> ()
        n249 = Enqueue Element(queue=w462, element=T2."import events", error in (no error)=w460) -> (queue out=w463:refnum<queue>, error out=w459:errorcluster)  [unwired: 1 in, 1 out]
      }
      event "pick event files": Mouse Up {
        # "promt user to select event files"
        n250 = event-data() -> ()  [unwired: 1 in, 7 out]
        n251 = call "event dialog"("error in"=w465) -> ("selected paths"=w469:path[], "cancelled"=w467:bool, "error out"=w466:errorcluster)  [unwired: 11 in, 1 out]
        n252 = local write "event files"(w469) -> ()
        n253 = Select(t=w465, s=w467, f=w466) -> (s? t:f=w464:errorcluster)
        n254 = Enqueue Element(queue=w471, element=T2."import events", error in (no error)=w464) -> (queue out=w472:refnum<queue>, error out=w468:errorcluster)  [unwired: 1 in, 1 out]
      }
      event "pick baseline files": Mouse Up {
        # "prompt user to select baseline files"
        n255 = event-data() -> ()  [unwired: 1 in, 7 out]
        n256 = call "base dialog"("error in"=w474) -> ("selected paths"=w478:path[], "cancelled"=w476:bool, "error out"=w475:errorcluster)  [unwired: 11 in, 1 out]
        n257 = local write "additional baseline files"(w478) -> ()
        n258 = Select(t=w474, s=w476, f=w475) -> (s? t:f=w473:errorcluster)
        n259 = Enqueue Element(queue=w480, element=T2."plot signals", error in (no error)=w473) -> (queue out=w481:refnum<queue>, error out=w477:errorcluster)  [unwired: 1 in, 1 out]
      }
      event "load defaults": Mouse Up {
        # "restore polynomial fit values to default\ngoing to read plot data state will reload the calibration constant from the event file if present"
        n260 = event-data() -> ()  [unwired: 1 in, 7 out]
        n261 = invoke on="subtract fraction" class="DigNum (strict)" method="Reinit To Default"(error in=w487) -> (error out=w492:errorcluster)  [unwired: 2 in, 2 out]
        n262 = invoke on="fit fraction" class="DigNum (strict)" method="Reinit To Default"(error in=w492) -> (error out=w491:errorcluster)  [unwired: 2 in, 2 out]
        n263 = invoke on="ignore first" class="DigNum (strict)" method="Reinit To Default"(error in=w491) -> (error out=w490:errorcluster)  [unwired: 2 in, 2 out]
        n264 = invoke on="fit order" class="DigNum (strict)" method="Reinit To Default"(error in=w490) -> (error out=w489:errorcluster)  [unwired: 2 in, 2 out]
        n265 = invoke on="ignore fraction" class="DigNum (strict)" method="Reinit To Default"(error in=w489) -> (error out=w488:errorcluster)  [unwired: 2 in, 2 out]
        n266 = invoke on="calibration constant" class="DigNum (strict)" method="Reinit To Default"(error in=w488) -> (error out=w484:errorcluster)  [unwired: 2 in, 2 out]
        n267 = Enqueue Element(queue=w486, element=T2."read plot data", error in (no error)=w484) -> (queue out=w482:refnum<queue>, error out=w483:errorcluster)  [unwired: 1 in, 1 out]
      }
      event "ignore first", "fit fraction", "ignore fraction", "calibration constant", "fit order", "subtract fraction": Value Change {
        n268 = event-data() -> ()  [unwired: 1 in, 5 out]
        n269 = Enqueue Element(queue=w494, element=T2."plot signals", error in (no error)=w495) -> (queue out=w497:refnum<queue>, error out=w496:errorcluster)  [unwired: 1 in, 1 out]
      }
      event "pick baseline": Mouse Up {
        w506 = u64 2082844800  # 01Jan1970, UTC
        # "use the currently selected signal as the baseline"
        n270 = event-data() -> ()  [unwired: 1 in, 7 out]
        n271 = local read "event"() -> (w503:string)
        n272 = local write "auto baseline"(FALSE ("auto baseline")) -> ()
        n273 = local write "baseline"(w503) -> ()
        n274 = Decimal String To Number(string=w503) -> (number=w507:i32)  [unwired: 2 in, 1 out]
        n275 = Add(x=w507, y=w506) -> (x+y=w505:u64)
        n276 = To Time Stamp(1:w505) -> (0:w504:timestamp)
        n277 = local write "baseline time"(w504) -> ()
        n278 = Enqueue Element(queue=w501, element=T2."plot signals", error in (no error)=w499) -> (queue out=w502:refnum<queue>, error out=w498:errorcluster)  [unwired: 1 in, 1 out]
      }
      event "auto baseline": Value Change {
        n279 = event-data() -> ("NewVal"=w513:bool)  [unwired: 1 in, 4 out]
        n280 = case shown="True" w513 {
          tunnel: w512 -> [w514 w519]
          tunnel: w511 -> [w515 w518]
          tunnel: [w515 w517] -> w510
          tunnel: [w514 w516] -> w509
          frame False {
          }
          frame True {
            n281 = Enqueue Element(queue=w518, element=T2."plot signals", error in (no error)=w519) -> (queue out=w517:refnum<queue>, error out=w516:errorcluster)  [unwired: 1 in, 1 out]
          }
        }
      }
      event "load": Mouse Up {
        # "load filter set from file"
        n282 = event-data() -> ()  [unwired: 1 in, 7 out]
        n283 = call "load filter"("error in"=w536) -> ("selected path"=w524:path, "error out"=w525:errorcluster)  [unwired: 11 in, 2 out]
        n284 = Get File Size(file=w524, error in=w525) -> (refnum out=w522:refnum<file>, 0:w523:errorcluster)  [unwired: 1 out]
        n285 = Read from Binary File(5:T6 {"fragment"="", "criteria"=[], "operator"=""} ("Cluster"), 8:w523, 9:T5."little-endian" ("byte order (0:big-endian, network order)"), 10:-1 ("count (1)"), 11:w522) -> (0:w532:errorcluster, 2:w534:T1, 3:w533:refnum<file>)  [unwired: 1 in, 1 out]
        n286 = local write "filter"(w534) -> ()
        n287 = Close File(refnum=w533, error in=w532) -> (error out=w528:errorcluster)  [unwired: 1 out]
        n288 = Enqueue Element(queue=w531, element=T2."filter events", error in (no error)=w528) -> (queue out=w530:refnum<queue>, error out=w527:errorcluster)  [unwired: 1 in, 1 out]
      }
      event "save": Mouse Up {
        # "save filter set to file"
        n289 = event-data() -> ()  [unwired: 1 in, 7 out]
        n290 = call "save filter"("error in"=w551) -> ("selected path"=w550:path, "error out"=w549:errorcluster)  [unwired: 11 in, 2 out]
        n291 = Strip Path(path=w550) -> (stripped path=w541:path, name=w543:string)
        n292 = Concatenate Strings(w543, ".tcl" ("string")) -> (w540:string)
        n293 = Build Path(base path=w541, name or relative path=w540) -> (appended path=w539:path)
        n294 = local read "filter"() -> (w546:T1)
        n295 = Write to Binary File(file (use dialog)=w539, data=w546, error in=w549, 5:FALSE ("prepend array or string size? (T)"), 9:T5."little-endian" ("byte order (0:big-endian, network order)")) -> (refnum out=w548:refnum<file>, error out=w547:errorcluster)  [unwired: 1 in, 1 out]
        n296 = Close File(refnum=w548, error in=w547) -> (error out=w545:errorcluster)  [unwired: 1 out]
      }
    }
    n297 = Unbundle By Name(w348) -> ("status"=w349:bool)
    n298 = local read "stop"() -> (w343:bool)
    n299 = Or(x=w349, y=w343) -> (x .or. y?=w344:bool)
  }
  n300 = Release Queue(queue=w14, error in (no error)=w13) -> (error out=w12:errorcluster)  [unwired: 1 in, 2 out]
  n301 = Merge Errors(w12, w11) -> (→"error out":errorcluster)
